vi "Advance past next JSON Value.vi"(7 "JSON":string, 9 "Offset":i32) -> (1 "Offset out":i32, 2 "Value start":i32, 3 "State":T1=enum."Value end")   [LabVIEW 2017, in "JSONtext.lvlib"]
uses:
  JSONtext.lvlib
  Parsing State.ctl
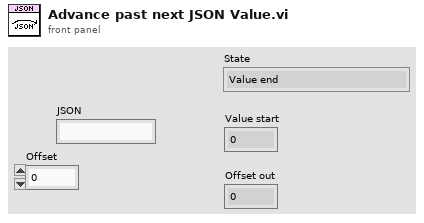
[diagram p1: front panel]
types:
  T1 = typedef "JSONtext.lvlib/Parsing State.ctl" = enum16{"Parser Error", "Object", "Array", "String", "Number/Other", "Leading Whitespace", "Object end", "Array end", "Value end"}
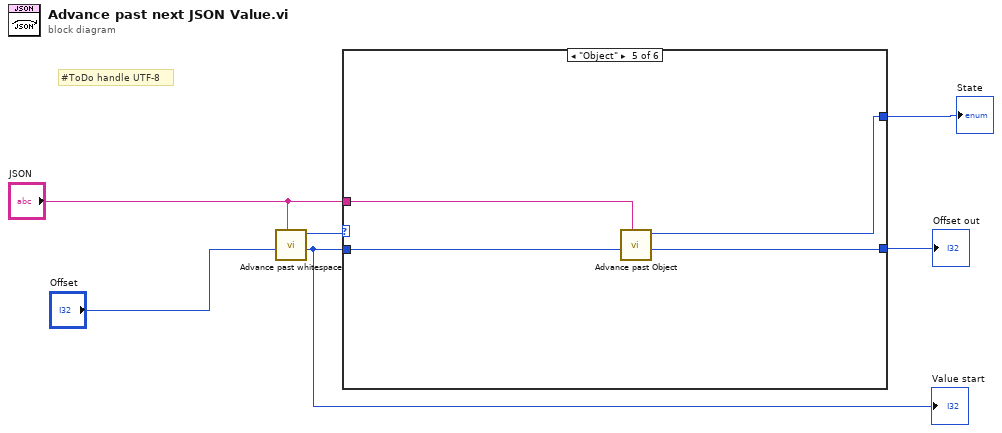
[diagram p0: block diagram]
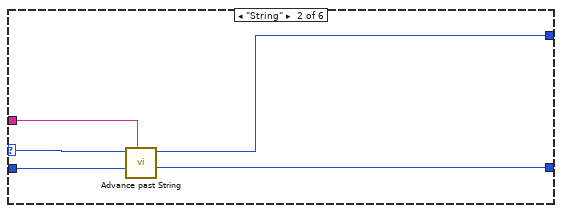
[diagram p3: hidden frame]
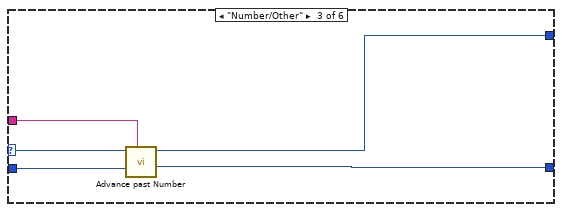
[diagram p4: hidden frame]
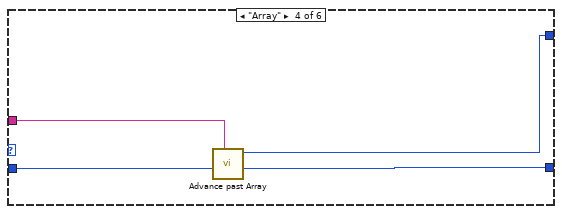
[diagram p5: hidden frame]
diagram:
  # "#ToDo handle UTF-8"
  n1 = call "Advance past whitespace.vi"("JSON"="JSON", "Offset"="Offset") -> ("Offset of first non-whitespace"=w1:i32, "Parser State"=w5:T1)  [unwired: 8 in]
  "Value start" <- w1
  n2 = case shown="\"Object\"" w5 {
    selector: w5 -> [w7 w12 w17 _ _ w27]
    tunnel: "JSON" -> [_ w13 w18 w19 w23 _]
    tunnel: w1 -> [w8 w11 w16 w20 w26 w28]
    tunnel: [w8 w10 w15 w21 w24 w28] -> w4
    tunnel: [w7 w9 w14 w22 w25 w27] -> w3
    frame "Parser Error", Default {
    }
    frame "String" {
      n3 = call "Advance past String.vi"("JSON"=w13, "Offset"=w11, "State in"=w12) -> ("Offset past match"=w10:i32, "State"=w9:T1)  [unwired: 6 in, 1 out]
    }
    frame "Number/Other" {
      n4 = call "Advance past Number.vi"("JSON"=w18, "Offset (0)"=w16, "Parser State in"=w17) -> ("Offset past match"=w15:i32, "Parser State"=w14:T1)  [unwired: 5 in, 2 out]
    }
    frame "Array" {
      n5 = call "Advance past Array.vi"("JSON"=w19, "Offset"=w20) -> ("Offset past Array"=w21:i32, "State"=w22:T1)  [unwired: 6 in, 2 out]
    }
    frame "Object" {
      n6 = call "Advance past Object.vi"("JSON"=w23, "Offset"=w26) -> ("Offset past Object"=w24:i32, "State"=w25:T1)  [unwired: 7 in, 1 out]
    }
    frame "Value end" {
      # "null, true, etc."
    }
  }
  "State" <- w3
  "Offset out" <- w4
